vi "changeROI.vi"(0 "FakeCamera in":refnum<class "MoveDataFile.lvclass">, 7 "Seperator":string, 9 "value":string, 11 "error in (no error)":errorcluster) -> (4 "FakeCamera out":refnum<class "MoveDataFile.lvclass">, 6 "output cluster":T1, 8 "value":dbl, 10 "Command out":string, 15 "error out":errorcluster)   [LabVIEW 2011, in "MoveDataFile.lvclass"]
uses:
  MoveDataFile.lvclass
  Program Files (x86)/National Instruments/LabVIEW 2011/resource/objmgr/imaqdx.rc
  <vilib>/vision/driver/NI_Vision_Acquisition_Software.lvlib
  shared/CompressAndUpdate(Poly)/CompressAndUpdate(Numeric).vi
  Point Grey Camera/subVis/ROI_TypDef.ctl
panel:
  out "output array":u32[](array[numeric])
  out "Y Resolution":i32
  out "X Resolution":i32
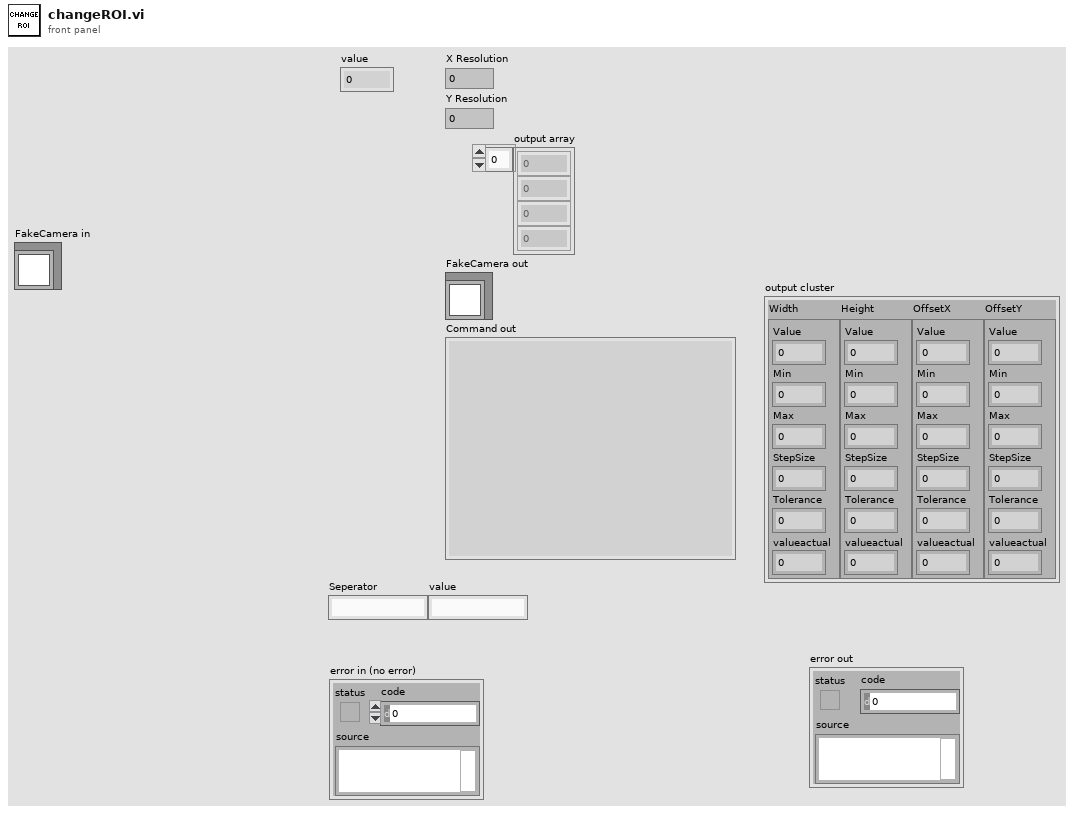
[diagram p1: front panel]
types:
  T1 = typedef "ROI_TypDef.ctl" = cluster{"Width":cluster{"Value":dbl, "Min":dbl, "Max":dbl, "StepSize":dbl, "Tolerance":dbl, "valueactual":dbl}, "Height":cluster{"Value":dbl, "Min":dbl, "Max":dbl, "StepSize":dbl, "Tolerance":dbl, "valueactual":dbl}, "OffsetX":cluster{"Value":dbl, "Min":dbl, "Max":dbl, "StepSize":dbl, "Tolerance":dbl, "valueactual":dbl}, "OffsetY":cluster{"Value":dbl, "Min":dbl, "Max":dbl, "StepSize":dbl, "Tolerance":dbl, "valueactual":dbl}}
  T2 = typedef "IMAQdx.ctl" = refnum<k21>
  T3 = typedef "Image Type" = u32
  T4 = typedef "CamAtributes_TypDEf.ctl" = cluster{"Gain":string, "Shutter":string, "TriggerDelay":string, "TriggerMode":string, "ROI Width":string, "ROI Height":string, "ROI OffsetX":string, "ROI OffsetY":string}
  T5 = typedef "Comparison.ctl" = enum16{"Greater", "Smaller", "Equal"}
  T6 = typedef "IMAQ Image.ctl" = refnum<image>
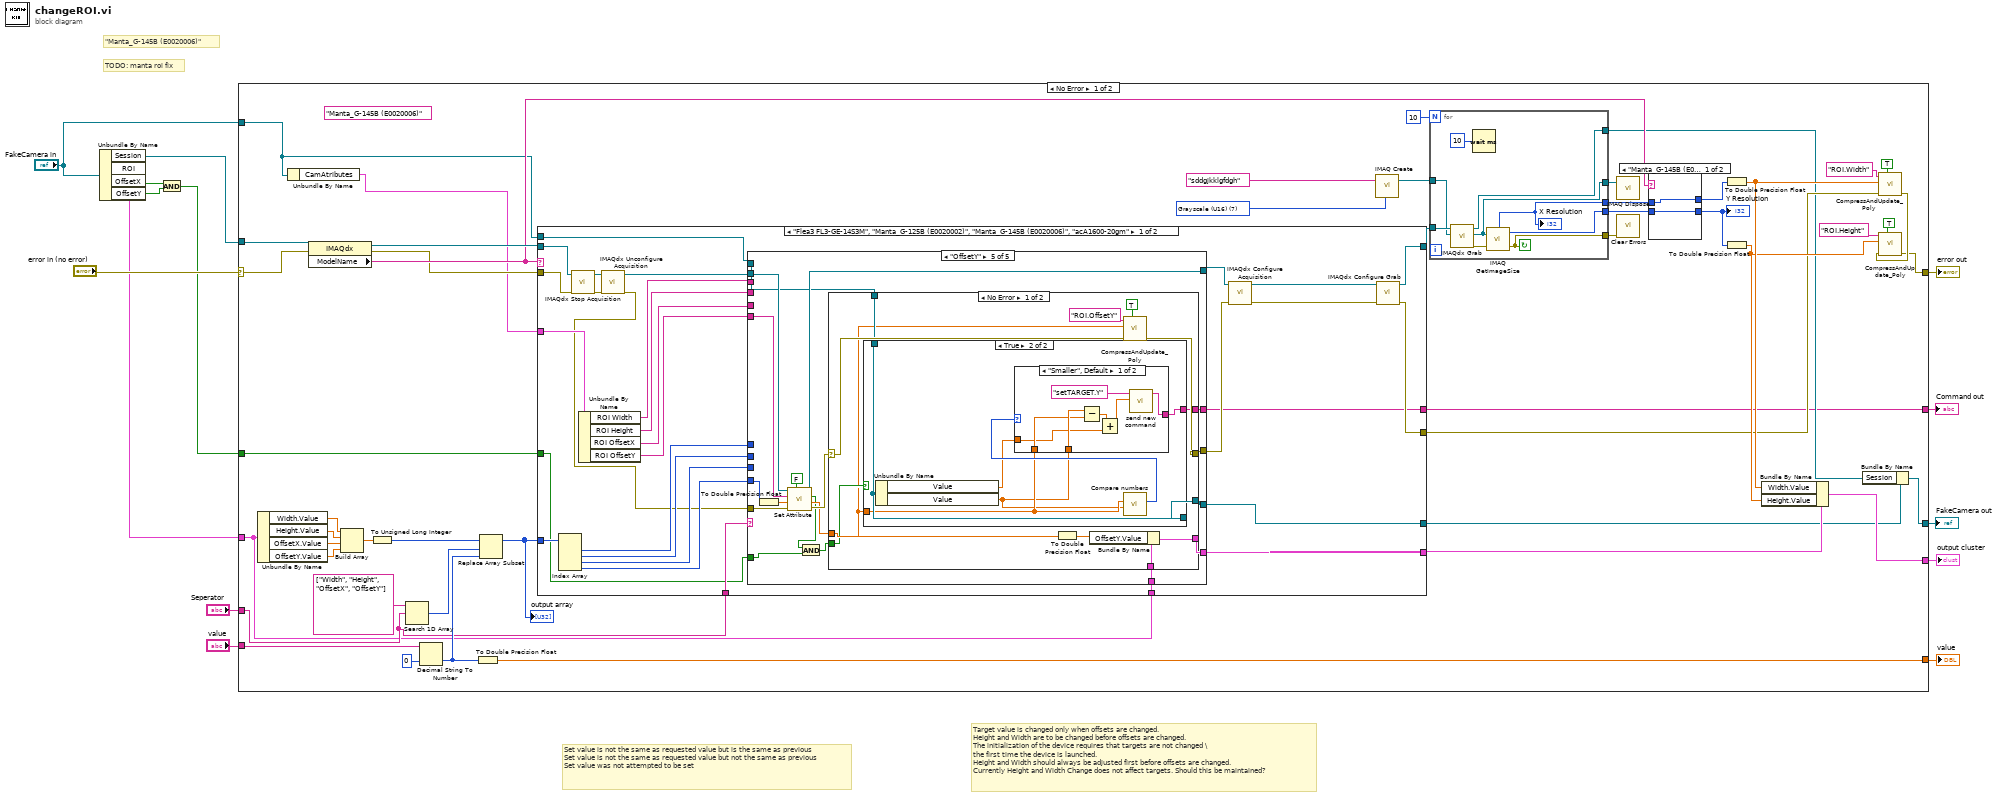
[diagram p0: block diagram]
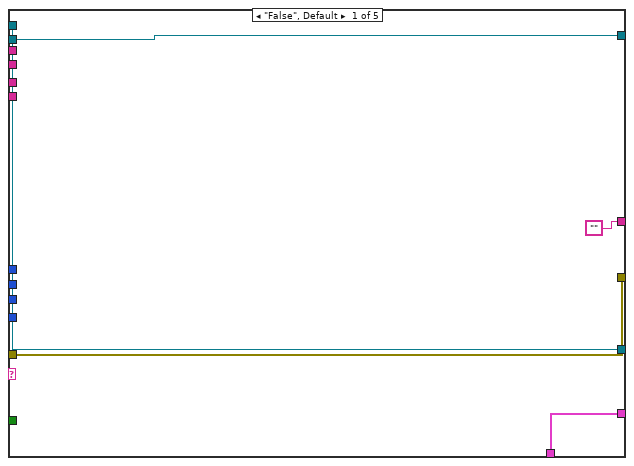
[diagram p3: hidden frame]
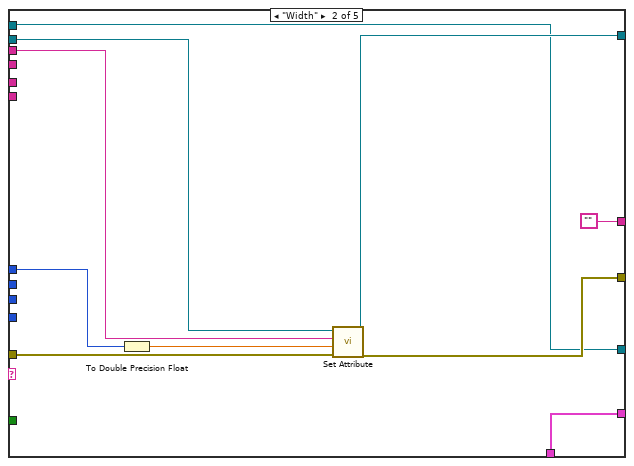
[diagram p4: hidden frame]
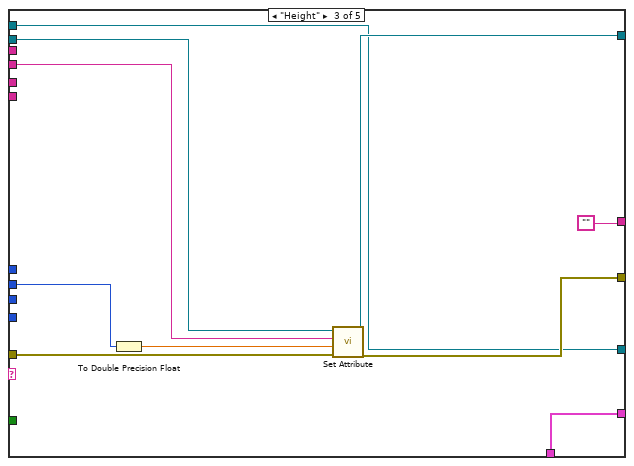
[diagram p5: hidden frame]
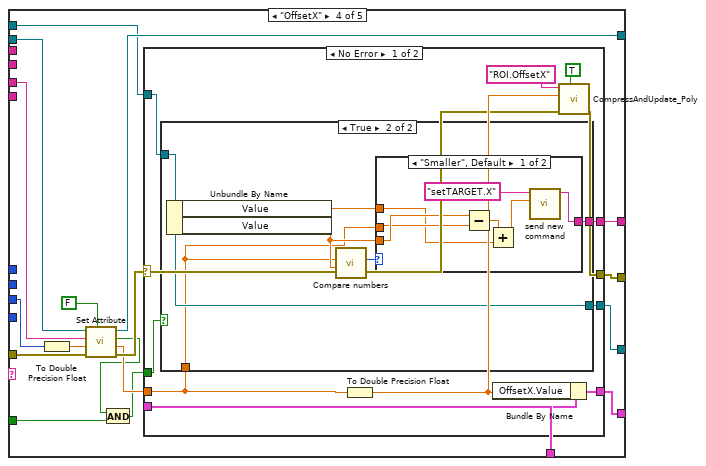
[diagram p6: hidden frame]
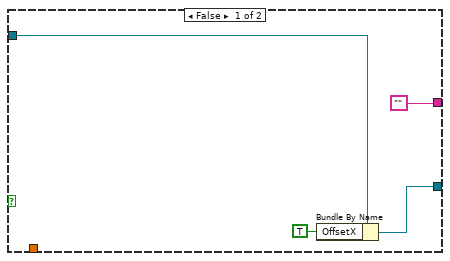
[diagram p7: hidden frame]
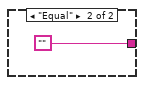
[diagram p8: hidden frame]
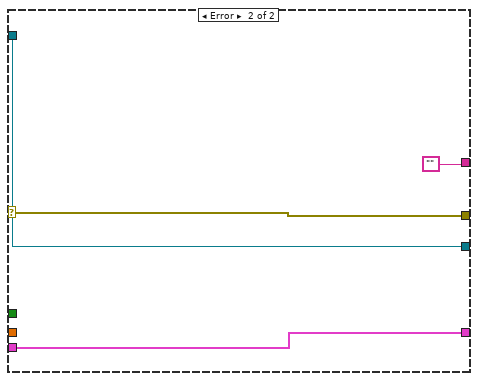
[diagram p9: hidden frame]
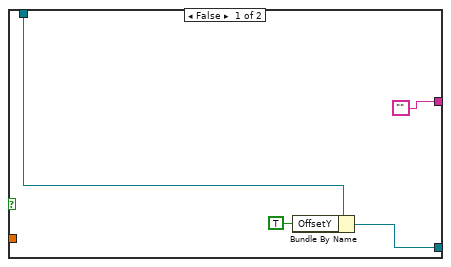
[diagram p10: hidden frame]
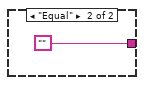
[diagram p11: hidden frame]
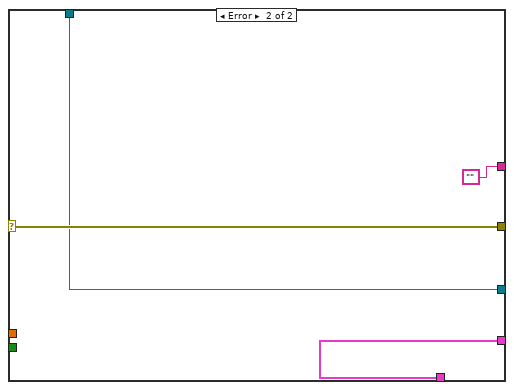
[diagram p12: hidden frame]
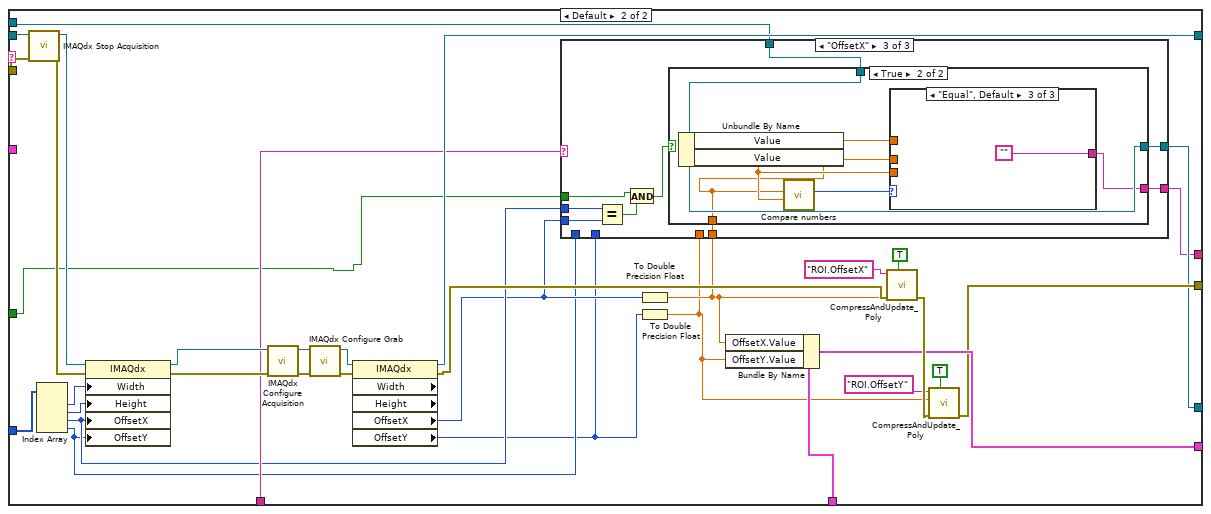
[diagram p13: hidden frame]
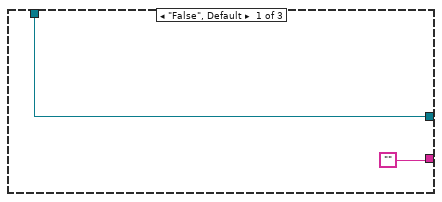
[diagram p14: hidden frame]
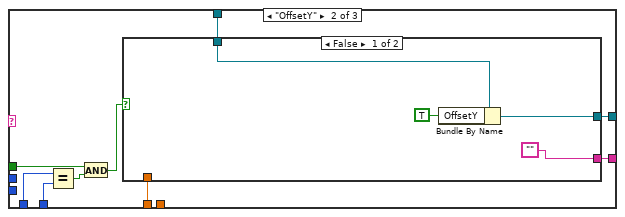
[diagram p15: hidden frame]
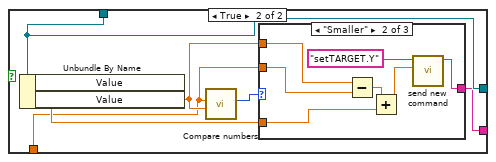
[diagram p16: hidden frame]
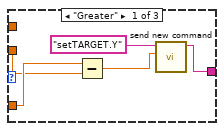
[diagram p17: hidden frame]
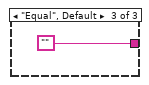
[diagram p18: hidden frame]
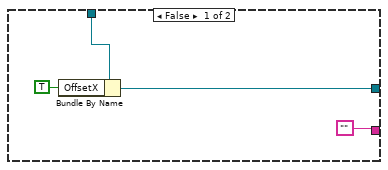
[diagram p19: hidden frame]
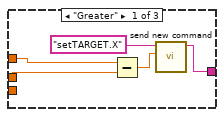
[diagram p20: hidden frame]
diagram:
  # "Target value is changed only when offsets are changed.\nHeight and Width are to be changed before offsets are changed.\nThe initialization of the device requires that targets are not changed \\\nthe first time the device is launched. \nHeight and Width should always be adjusted first before offsets are changed.\nCurrently Height and Width Change does not affect targets. Should this be maintained?"
  # "Set value is not the same as requested value but is the same as previous\nSet value is not the same as requested value but not the same as previous\nSet value was not attempted to be set"
  # "TODO: manta roi fix"
  # "\"Manta_G-145B (E0020006)\""
  n1 = Unbundle By Name("FakeCamera in") -> ("Session"=w7:T2, "ROI"=w8:T1, "OffsetX"=w5:bool, "OffsetY"=w6:bool)
  n2 = And(x=w5, y=w6) -> (x .and. y?=w4:bool)
  n3 = case shown="No Error" "error in (no error)" {
    selector: "error in (no error)" -> [w29 w338]
    tunnel: w7 -> [w30 _]
    tunnel: "Seperator" -> [w25 _]
    tunnel: "value" -> [w61 _]
    tunnel: w8 -> [w24 w337]
    tunnel: [w55 w337] -> w12
    tunnel: [w22 w338] -> w11
    tunnel: [w51 _] -> w9
    tunnel: w4 -> [w21 _]
    tunnel: "FakeCamera in" -> [w20 w336]
    tunnel: [w16 w336] -> w2
    tunnel: [w15 ""] -> w1
    frame No Error {
      (unwired) "Manta_G-145B (E0020006)"
      w41 = T3 7 items=["Grayscale (U8)", "Grayscale (I16)", "Grayscale (SGL)", "Complex (CSG)", "RGB (U32)", "HSL (U32)", "RGB (U64)", "Grayscale (U16)"] ("Image Type")
      n4 = Unbundle By Name(w24) -> ("Width.Value"=w60:dbl, "Height.Value"=w59:dbl, "OffsetX.Value"=w58:dbl, "OffsetY.Value"=w57:dbl)
      n5 = Unbundle By Name(w20) -> ("CamAtributes"=w19:T4)
      n6 = property class="IMAQdx"(reference=w30, error in=w29) -> (reference out=w37:T2, error out=w28:errorcluster, "ModelName"=w36:string)
      n7 = Build Array(w60, w59, w58, w57) -> (w56:dbl[])
      n8 = To Unsigned Long Integer(number=w56) -> (unsigned 32bit integer=w54:u32[])
      n9 = Search 1D Array(1D array=string[] ["Width", "Height", "OffsetX", "OffsetY"] ("Seperator"), element=w25) -> (index of element=w53:i32)  [unwired: 1 in]
      n10 = Decimal String To Number(string=w61, default (0L)=u32 0 ("default (0 I32)")) -> (number=w52:u32)  [unwired: 1 in, 1 out]
      n11 = To Double Precision Float(number=w52) -> (double precision float=w51:dbl)
      n12 = Replace Array Subset(array=w54, new element=w52, index=w53) -> (w31:u32[])
      "output array" <- w31
      n13 = case shown="\"Flea3 FL3-GE-14S3M\", \"Manta_G-125B (E0020002)\", \"Manta_G-145B (E0020006)\", \"acA1600-20gm\"" w36 {
        tunnel: w37 -> [w83 w249]
        tunnel: w31 -> [w96 w254]
        tunnel: w28 -> [w82 w247]
        tunnel: [w77 w237] -> w27
        tunnel: [w76 w250] -> w44
        tunnel: w19 -> [w95 _]
        tunnel: w25 -> [w92 w236]
        tunnel: w24 -> [w85 w240]
        tunnel: [w84 w239] -> w23
        tunnel: w21 -> [w72 w235]
        tunnel: w20 -> [w71 w231]
        tunnel: [w70 w230] -> w18
        tunnel: [w69 w229] -> w15
        frame "Flea3 FL3-GE-14S3M", "Manta_G-125B (E0020002)", "Manta_G-145B (E0020006)", "acA1600-20gm" {
          n14 = Index Array(array=w96) -> (element #1=w93:u32, element #2=w91:u32, element #3=w88:u32, element #4=w87:u32)  [unwired: 4 in]
          n15 = call <vilib>:"IMAQdx Stop Acquisition.vi"("error in"=w82, "Session In"=w83) -> ("error out"=w75:errorcluster, "Session Out"=w74:T2)  [unwired: 8 in]
          n16 = Unbundle By Name(w95) -> ("ROI Width"=w94:string, "ROI Height"=w90:string, "ROI OffsetX"=w89:string, "ROI OffsetY"=w86:string)
          n17 = call <vilib>:"IMAQdx Unconfigure Acquisition.vi"("error in"=w75, "Session In"=w74) -> ("error out"=w73:errorcluster, "Session Out"=w68:T2)  [unwired: 8 out]
          n18 = case shown="\"OffsetY\"" w92 {
            tunnel: w68 -> [w101 w111 w121 w139 w191]
            tunnel: w94 -> [_ w110 _ _ _]
            tunnel: w93 -> [_ w109 _ _ _]
            tunnel: w73 -> [w100 w108 w120 w138 w190]
            tunnel: [w101 w107 w119 w137 w189] -> w79
            tunnel: [w100 w106 w118 w132 w184] -> w78
            tunnel: w91 -> [_ _ w115 _ _]
            tunnel: w90 -> [_ _ w117 _ _]
            tunnel: w89 -> [_ _ _ w136 _]
            tunnel: w88 -> [_ _ _ w135 _]
            tunnel: w87 -> [_ _ _ _ w187]
            tunnel: w86 -> [_ _ _ _ w188]
            tunnel: w85 -> [w99 w105 w116 w133 w186]
            tunnel: [w99 w105 w116 w134 w185] -> w84
            tunnel: w72 -> [_ _ _ w126 w178]
            tunnel: w71 -> [w98 w104 w114 w130 w182]
            tunnel: [w98 w104 w114 w129 w181] -> w70
            tunnel: ["" "" "" w124 w176] -> w69
            frame "False", Default {
            }
            frame "Width" {
              n19 = To Double Precision Float(number=w109) -> (double precision float=w102:dbl)
              n20 = call "Set Attribute.vi"("error in (no error)"=w108, "Value"=w102, "Attribute Name"=w110, "Session In"=w111) -> ("error out"=w106:errorcluster, "IMAQdx Session out"=w107:T2)  [unwired: 4 in, 2 out]
            }
            frame "Height" {
              n21 = To Double Precision Float(number=w115) -> (double precision float=w112:dbl)
              n22 = call "Set Attribute.vi"("error in (no error)"=w120, "Value"=w112, "Attribute Name"=w117, "Session In"=w121) -> ("error out"=w118:errorcluster, "IMAQdx Session out"=w119:T2)  [unwired: 4 in, 2 out]
            }
            frame "OffsetX" {
              n23 = To Double Precision Float(number=w135) -> (double precision float=w128:dbl)
              n24 = call "Set Attribute.vi"("coerce if out of range"=FALSE, "error in (no error)"=w138, "Value"=w128, "Attribute Name"=w136, "Session In"=w139) -> ("error out"=w131:errorcluster, "Value Out"=w127:dbl, "Value Changed?"=w122:bool, "IMAQdx Session out"=w137:T2)  [unwired: 3 in]
              n25 = And(x=w122, y=w126) -> (x .and. y?=w125:bool)
              n26 = case shown="No Error" w131 {
                selector: w131 -> [w146 w173]
                tunnel: w127 -> [w141 _]
                tunnel: [w151 w172] -> w134
                tunnel: w133 -> [w144 w172]
                tunnel: [w148 w173] -> w132
                tunnel: w125 -> [w145 _]
                tunnel: w130 -> [w143 w171]
                tunnel: [w142 w171] -> w129
                tunnel: [w140 ""] -> w124
                frame No Error {
                  n27 = case shown="True" w145 {
                    tunnel: w143 -> [w152 w158]
                    tunnel: [w154 w158] -> w142
                    tunnel: w141 -> [_ w157]
                    tunnel: ["" w156] -> w140
                    frame False {
                      n28 = Bundle By Name(cluster=w152, "OffsetX"=TRUE) -> (w154:refnum<class "MoveDataFile.lvclass">)
                    }
                    frame True {
                      n29 = Unbundle By Name(w158) -> ("Value"=w160:dbl, "Value"=w159:dbl)
                      n30 = call "Compare numbers.vi"("Prev"=w159, "New"=w157) -> ("comparison"=w161:T5)  [unwired: 9 in]
                      n31 = case shown="\"Smaller\", Default" w161 {
                        tunnel: w160 -> [w165 _]
                        tunnel: w157 -> [w167 _]
                        tunnel: [w162 ""] -> w156
                        tunnel: w159 -> [w168 _]
                        frame "Smaller", Default {
                          n32 = Subtract(x=w168, y=w167) -> (x-y=w166:dbl)
                          n33 = Add(x=w166, y=w165) -> (x+y=w163:dbl)
                          n34 = call "send new command.vi"("number"=w163, "string"="setTARGET.X") -> ("String"=w162:string)  [unwired: 9 in]
                        }
                        frame "Equal" {
                        }
                      }
                    }
                  }
                  n35 = To Double Precision Float(number=w141) -> (double precision float=w147:dbl)
                  n36 = Bundle By Name(cluster=w144, "OffsetX.Value"=w147) -> (w151:T1)
                  n37 = call-poly "CompressAndUpdate_Poly.vi"("force CVT update (false)"=TRUE, "error in"=w146, "Numeric"=w147, "command or variable name"="ROI.OffsetX") -> ("error out"=w148:errorcluster)  [unwired: 7 in]
                }
                frame Error {
                }
              }
            }
            frame "OffsetY" {
              n38 = To Double Precision Float(number=w187) -> (double precision float=w180:dbl)
              n39 = call "Set Attribute.vi"("coerce if out of range"=FALSE, "error in (no error)"=w190, "Value"=w180, "Attribute Name"=w188, "Session In"=w191) -> ("error out"=w183:errorcluster, "Value Out"=w179:dbl, "Value Changed?"=w174:bool, "IMAQdx Session out"=w189:T2)  [unwired: 3 in]
              n40 = And(x=w174, y=w178) -> (x .and. y?=w177:bool)
              n41 = case shown="No Error" w183 {
                selector: w183 -> [w197 w225]
                tunnel: w186 -> [w203 w224]
                tunnel: [w202 w224] -> w185
                tunnel: w179 -> [w201 _]
                tunnel: [w198 w225] -> w184
                tunnel: w177 -> [w196 _]
                tunnel: w182 -> [w195 w223]
                tunnel: [w194 w223] -> w181
                tunnel: [w192 ""] -> w176
                frame No Error {
                  n42 = To Double Precision Float(number=w201) -> (double precision float=w193:dbl)
                  n43 = case shown="True" w196 {
                    tunnel: w195 -> [w207 w213]
                    tunnel: [w205 w213] -> w194
                    tunnel: w193 -> [_ w210]
                    tunnel: ["" w208] -> w192
                    frame False {
                      n44 = Bundle By Name(cluster=w207, "OffsetY"=TRUE) -> (w205:refnum<class "MoveDataFile.lvclass">)
                    }
                    frame True {
                      n45 = Unbundle By Name(w213) -> ("Value"=w211:dbl, "Value"=w209:dbl)
                      n46 = call "Compare numbers.vi"("Prev"=w209, "New"=w210) -> ("comparison"=w212:T5)  [unwired: 9 in]
                      n47 = case shown="\"Smaller\", Default" w212 {
                        tunnel: w211 -> [w217 _]
                        tunnel: w210 -> [w219 _]
                        tunnel: [w214 ""] -> w208
                        tunnel: w209 -> [w220 _]
                        frame "Smaller", Default {
                          n48 = Subtract(x=w220, y=w219) -> (x-y=w218:dbl)
                          n49 = Add(x=w218, y=w217) -> (x+y=w215:dbl)
                          n50 = call "send new command.vi"("number"=w215, "string"="setTARGET.Y") -> ("String"=w214:string)  [unwired: 9 in]
                        }
                        frame "Equal" {
                        }
                      }
                    }
                  }
                  n51 = Bundle By Name(cluster=w203, "OffsetY.Value"=w193) -> (w202:T1)
                  n52 = call-poly "CompressAndUpdate_Poly.vi"("force CVT update (false)"=TRUE, "error in"=w197, "Numeric"=w193, "command or variable name"="ROI.OffsetY") -> ("error out"=w198:errorcluster)  [unwired: 7 in]
                }
                frame Error {
                }
              }
            }
          }
          n53 = call <vilib>:"IMAQdx Configure Acquisition.vi"("error in"=w78, "Session In"=w79) -> ("error out"=w80:errorcluster, "Session Out"=w81:T2)  [unwired: 8 in]
          n54 = call <vilib>:"IMAQdx Configure Grab.vi"("error in"=w80, "Session In"=w81) -> ("error out"=w77:errorcluster, "Session Out"=w76:T2)  [unwired: 8 out]
        }
        frame Default {
          n55 = call <vilib>:"IMAQdx Stop Acquisition.vi"("error in"=w247, "Session In"=w249) -> ("error out"=w246:errorcluster, "Session Out"=w248:T2)  [unwired: 8 in]
          n56 = Index Array(array=w254) -> (element #1=w257:u32, element #2=w256:u32, element #3=w234:u32, element #4=w228:u32)  [unwired: 4 in]
          n57 = property class="IMAQdx"(reference=w248, error in=w246, "Width"=w257, "Height"=w256, "OffsetX"=w234, "OffsetY"=w228) -> (reference out=w259:T2, error out=w253:errorcluster)
          n58 = call <vilib>:"IMAQdx Configure Acquisition.vi"("error in"=w253, "Session In"=w259) -> ("error out"=w252:errorcluster, "Session Out"=w258:T2)  [unwired: 8 in]
          n59 = call <vilib>:"IMAQdx Configure Grab.vi"("error in"=w252, "Session In"=w258) -> ("error out"=w251:errorcluster, "Session Out"=w255:T2)  [unwired: 8 out]
          n60 = property class="IMAQdx" props=["Width", "Height", "OffsetX", "OffsetY"](reference=w255, error in=w251) -> (reference out=w250:T2, error out=w238:errorcluster, "OffsetX"=w233:u32, "OffsetY"=w227:u32)  [unwired: 2 out]
          n61 = To Double Precision Float(number=w233) -> (double precision float=w232:dbl)
          n62 = To Double Precision Float(number=w227) -> (double precision float=w226:dbl)
          n63 = case shown="\"OffsetX\"" w236 {
            tunnel: w235 -> [_ w269 w300]
            tunnel: w234 -> [_ _ w302]
            tunnel: w233 -> [_ _ w301]
            tunnel: w231 -> [w260 w265 w297]
            tunnel: w232 -> [_ _ w296]
            tunnel: [w260 w264 w295] -> w230
            tunnel: ["" w263 w294] -> w229
            tunnel: w228 -> [_ w268 _]
            tunnel: w227 -> [_ w267 _]
            tunnel: w226 -> [_ w262 _]
            frame "False", Default {
            }
            frame "OffsetY" {
              n64 = Equal?(x=w268, y=w267) -> (x = y?=w270:bool)
              n65 = And(x=w269, y=w270) -> (x .and. y?=w266:bool)
              n66 = case shown="False" w266 {
                tunnel: w265 -> [w274 w277]
                tunnel: [w273 w277] -> w264
                tunnel: ["" w276] -> w263
                tunnel: w262 -> [_ w275]
                frame False {
                  n67 = Bundle By Name(cluster=w274, "OffsetY"=TRUE) -> (w273:refnum<class "MoveDataFile.lvclass">)
                }
                frame True {
                  n68 = Unbundle By Name(w277) -> ("Value"=w279:dbl, "Value"=w278:dbl)
                  n69 = call "Compare numbers.vi"("Prev"=w278, "New"=w275) -> ("comparison"=w280:T5)  [unwired: 9 in]
                  n70 = case shown="\"Smaller\"" w280 {
                    tunnel: w279 -> [w285 w289 _]
                    tunnel: w275 -> [w284 w291 _]
                    tunnel: [w281 w286 ""] -> w276
                    tunnel: w278 -> [_ w292 _]
                    frame "Greater" {
                      n71 = Subtract(x=w285, y=w284) -> (x-y=w283:dbl)
                      n72 = call "send new command.vi"("number"=w283, "string"="setTARGET.Y") -> ("String"=w281:string)  [unwired: 9 in]
                    }
                    frame "Smaller" {
                      n73 = Subtract(x=w292, y=w291) -> (x-y=w290:dbl)
                      n74 = Add(x=w290, y=w289) -> (x+y=w287:dbl)
                      n75 = call "send new command.vi"("number"=w287, "string"="setTARGET.Y") -> ("String"=w286:string)  [unwired: 9 in]
                    }
                    frame "Equal", Default {
                    }
                  }
                }
              }
            }
            frame "OffsetX" {
              n76 = Equal?(x=w302, y=w301) -> (x = y?=w299:bool)
              n77 = And(x=w300, y=w299) -> (x .and. y?=w298:bool)
              n78 = case shown="True" w298 {
                tunnel: w297 -> [w306 w309]
                tunnel: [w305 w309] -> w295
                tunnel: w296 -> [_ w308]
                tunnel: ["" w307] -> w294
                frame False {
                  n79 = Bundle By Name(cluster=w306, "OffsetX"=TRUE) -> (w305:refnum<class "MoveDataFile.lvclass">)
                }
                frame True {
                  n80 = Unbundle By Name(w309) -> ("Value"=w311:dbl, "Value"=w310:dbl)
                  n81 = call "Compare numbers.vi"("Prev"=w310, "New"=w308) -> ("comparison"=w312:T5)  [unwired: 9 in]
                  n82 = case shown="\"Equal\", Default" w312 {
                    tunnel: w311 -> [w317 w321 _]
                    tunnel: w308 -> [w316 w323 _]
                    tunnel: [w313 w318 ""] -> w307
                    tunnel: w310 -> [_ w324 _]
                    frame "Greater" {
                      n83 = Subtract(x=w317, y=w316) -> (x-y=w315:dbl)
                      n84 = call "send new command.vi"("number"=w315, "string"="setTARGET.X") -> ("String"=w313:string)  [unwired: 9 in]
                    }
                    frame "Smaller" {
                      n85 = Subtract(x=w324, y=w323) -> (x-y=w322:dbl)
                      n86 = Add(x=w322, y=w321) -> (x+y=w319:dbl)
                      n87 = call "send new command.vi"("number"=w319, "string"="setTARGET.X") -> ("String"=w318:string)  [unwired: 9 in]
                    }
                    frame "Equal", Default {
                    }
                  }
                }
              }
            }
          }
          n88 = Bundle By Name(cluster=w240, "OffsetX.Value"=w232, "OffsetY.Value"=w226) -> (w239:T1)
          n89 = call-poly "CompressAndUpdate_Poly.vi"("force CVT update (false)"=TRUE, "error in"=w238, "Numeric"=w232, "command or variable name"="ROI.OffsetX") -> ("error out"=w245:errorcluster)  [unwired: 7 in]
          n90 = call-poly "CompressAndUpdate_Poly.vi"("force CVT update (false)"=TRUE, "error in"=w245, "Numeric"=w226, "command or variable name"="ROI.OffsetY") -> ("error out"=w237:errorcluster)  [unwired: 7 in]
        }
      }
      n91 = call "IMAQ Create"("Image Name"="sddgjkklgfdgh", "Image Type"=w41) -> ("New Image"=w43:T6)  [unwired: 3 in, 1 out]
      n92 = for {
        N: 10 -> [_]
        tunnel: w44 -> [w334]
        tunnel: w43 -> [w333]
        tunnel: [w332] -> w40
        tunnel: [w331] -> w17
        tunnel: [w330] -> w35
        tunnel: [w329] -> w33
        tunnel: [w328] -> w39
        stop <- w328 continue-if-true
        n93 = call <vilib>:"IMAQdx Grab.vi"("Image In"=w333, "Session In"=w334) -> ("error out"=w326:errorcluster, "Image Out"=w332:T6, "Session Out"=w331:T2)  [unwired: 6 in, 1 out]
        n94 = Wait (ms)(milliseconds to wait=u32 10) -> ()  [unwired: 1 out]
        n95 = call "IMAQ GetImageSize"("Image"=w332, "error in (no error)"=w326) -> ("Y Resolution"=w329:i32, "X Resolution"=w330:i32, "error out"=w328:errorcluster)  [unwired: 2 in]
        "X Resolution" <- w330
      }
      n96 = call "IMAQ Dispose"("Image"=w40) -> ()  [unwired: 5 in, 1 out]
      n97 = call <vilib>:"Clear Errors.vi"("error in (no error)"=w39) -> ()  [unwired: 6 in, 1 out]
      n98 = case shown="\"Manta_G-145B (E0020006)\", \"acA1600-20gm\"" w36 {
        tunnel: [w65 w67] -> w34
        tunnel: [w64 w66] -> w32
        tunnel: w35 -> [w65 w67]
        tunnel: w33 -> [w64 w66]
        frame "Manta_G-145B (E0020006)", "acA1600-20gm" {
        }
        frame Default {
        }
      }
      "Y Resolution" <- w32
      n99 = To Double Precision Float(number=w34) -> (double precision float=w49:dbl)
      n100 = To Double Precision Float(number=w32) -> (double precision float=w47:dbl)
      n101 = Bundle By Name(cluster=w23, "Width.Value"=w49, "Height.Value"=w47) -> (w55:T1)
      n102 = Bundle By Name(cluster=w18, "Session"=w17) -> (w16:refnum<class "MoveDataFile.lvclass">)
      n103 = call-poly "CompressAndUpdate_Poly.vi"("force CVT update (false)"=TRUE, "error in"=w27, "Numeric"=w49, "command or variable name"="ROI.Width") -> ("error out"=w26:errorcluster)  [unwired: 7 in]
      n104 = call-poly "CompressAndUpdate_Poly.vi"("force CVT update (false)"=TRUE, "error in"=w26, "Numeric"=w47, "command or variable name"="ROI.Height") -> ("error out"=w22:errorcluster)  [unwired: 7 in]
    }
    frame Error {
    }
  }
  "output cluster" <- w12
  "error out" <- w11
  "value" <- w9
  "FakeCamera out" <- w2
  "Command out" <- w1
